vi "停止.vi"(8 "error in (no error)":errorcluster) -> (0 "error out":errorcluster)   [LabVIEW 2020, in "输出轴伺服.lvlib"]
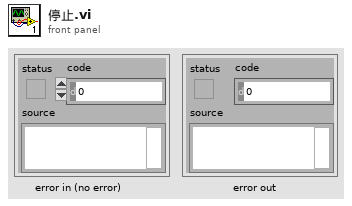
[diagram p1: front panel]
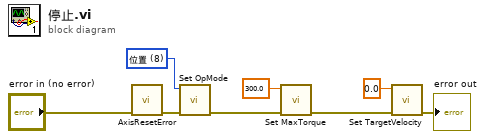
[diagram p0: block diagram]
diagram:
  w4 = u32 8 items=["位置"=8, "速度"=9, "扭矩"=10] ("Value")
  n1 = call "AxisResetError.vi"("error in (no error)"="error in (no error)") -> ("error out"=w2:errorcluster)  [unwired: 10 in]
  n2 = call "Set OpMode.vi"("error in (no error)"=w2, "Value"=w4) -> ("error out"=w1:errorcluster)  [unwired: 9 in]
  n3 = call "Set MaxTorque.vi"("error in (no error)"=w1, "Value"=sgl 300.0) -> ("error out"=w8:errorcluster)  [unwired: 9 in]
  n4 = call "Set TargetVelocity.vi"("error in (no error)"=w8, "Value"=sgl 0.0) -> ("error out"=→"error out":errorcluster)  [unwired: 9 in]
